vi "Gecko anesthesia specs.vi"(0 "ear folder path":path) -> ()   [LabVIEW 2010]
panel:
  in  "End & don't save":bool
  in  "conc of anesth":string="Concentration of anesthesia delivered (ml/mg): XX"
  in  "tag #":string="Animal number: XX"
  in  "mass":string="Mass (g): XX"
  in  "Length":string="Length (mm): XX"
  in  "method of anesth adminin":string="Method of anesthesia adminisration: XX"
  in  "comments":string="Comments: XX"
  in  "amt of anesth":string="Amount of anesthesia delivered (ml): XX"
  in  "OK; end & save":bool
  in  "anesthetic":string="Anesthetic: XX"
  in  "Sex":string="Sex: XX"
  in  "Animal species":string="Species: XX"
  in  "time of anesth":string="Time of anesthesia administration: XX"
  # "HARD SPECS:"
  # "ANESTHESIA:"
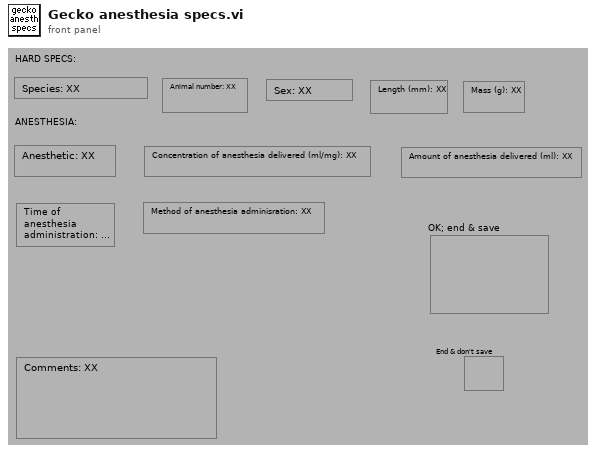
[diagram p1: front panel]
types:
  T1 = cluster{i32, i32, i32, i32, i32, i32, i32, i32, i32}
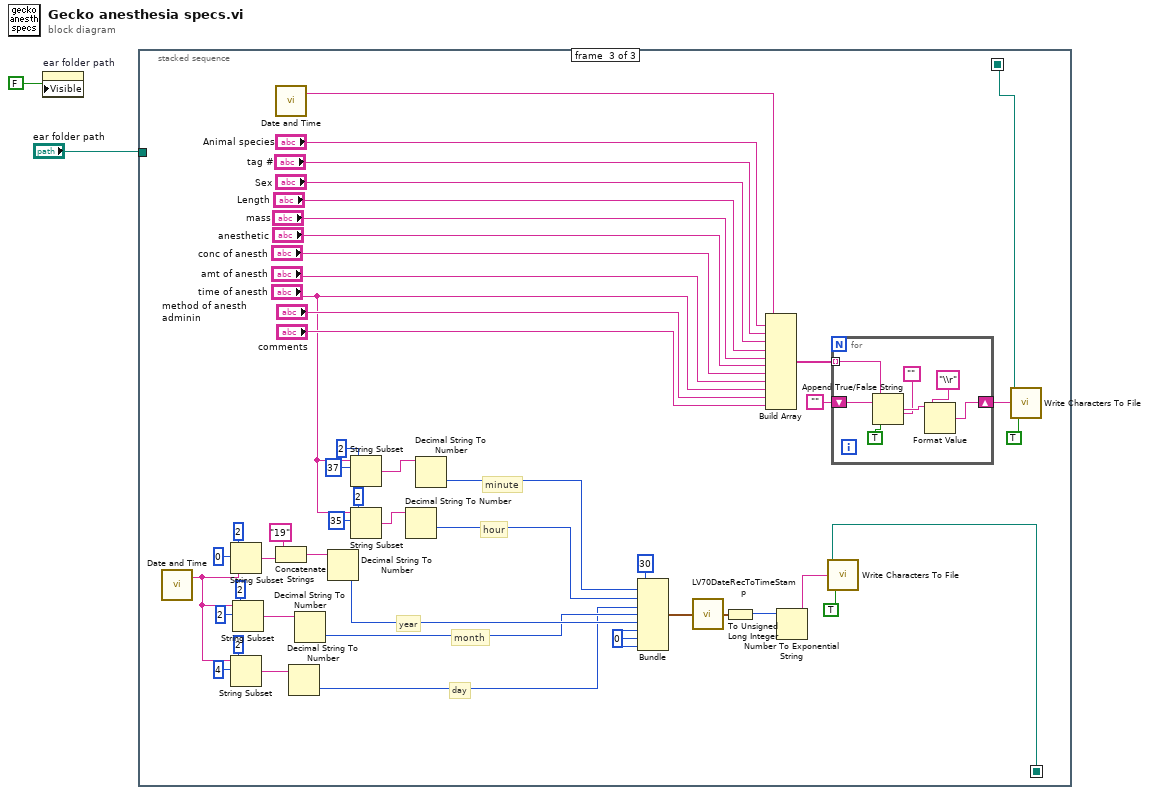
[diagram p0: block diagram]
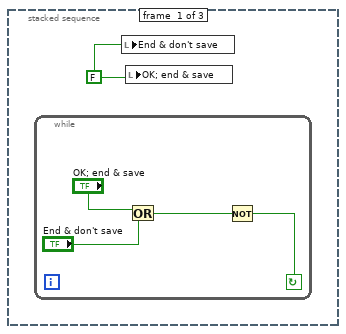
[diagram p2: hidden frame]
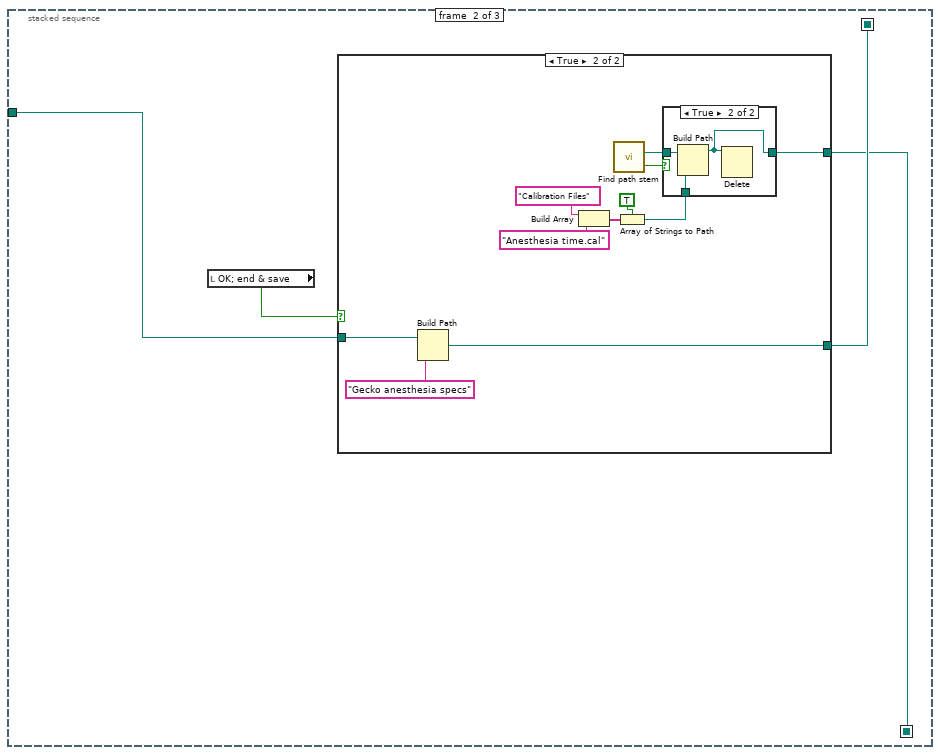
[diagram p3: hidden frame]
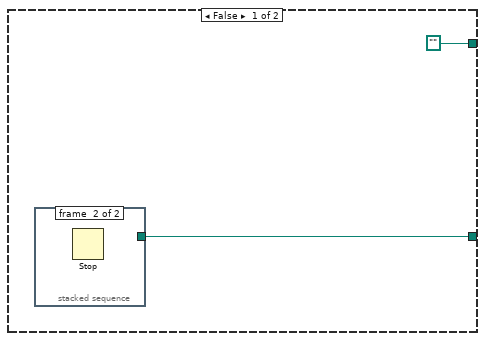
[diagram p4: hidden frame]
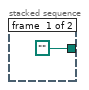
[diagram p5: hidden frame]
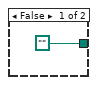
[diagram p6: hidden frame]
diagram:
  n1 = property on="ear folder path" class="Path"("Visible"=FALSE) -> ()  [unwired: 2 in, 2 out]
  n2 = stacked-sequence {
    seq-local: [_ w9 _] -> [_ _ w31]
    seq-local: [_ w8 _] -> [_ _ w34]
    tunnel: "ear folder path" -> [_ w10 _]
    frame #0 {
      w3 = FALSE
      n3 = while {
        stop <- w7 continue-if-true
        n4 = Or(x="OK; end & save", y="End & don't save") -> (x .or. y?=w6:bool)
        n5 = Not(x=w6) -> (.not. x?=w7:bool)
      }
      n6 = local write "End & don't save"(w3) -> ()
      n7 = local write "OK; end & save"(w3) -> ()
    }
    frame #1 {
      n8 = local read "OK; end & save"() -> (w11:bool)
      n9 = case shown="True" w11 {
        tunnel: w10 -> [_ w24]
        tunnel: [w13 w23] -> w9
        tunnel: [path "" w15] -> w8
        frame False {
          n10 = stacked-sequence {
            tunnel: [path "" _] -> w13
            frame #0 {
            }
            frame #1 {
              n11 = Stop() -> ()  [unwired: 1 out]
            }
          }
        }
        frame True {
          n12 = Build Path(base path=w24, name or relative path="Gecko anesthesia specs") -> (appended path=w23:path)
          n13 = Build Array("Calibration Files", "Anesthesia time.cal") -> (w19:string[])
          n14 = call "Find path stem.vi"() -> ("PASS/FAIL"=w17:bool, "Path stem."=w18:path)
          n15 = Array of Strings to Path(0:w19, 1:TRUE) -> (2:w16:path)
          n16 = case shown="True" w17 {
            tunnel: w18 -> [_ w29]
            tunnel: w16 -> [_ w28]
            tunnel: [path "" w27] -> w15
            frame False {
            }
            frame True {
              n17 = Build Path(base path=w29, name or relative path=w28) -> (appended path=w27:path)
              n18 = Delete(path (use dialog)=w27) -> ()  [unwired: 1 in, 6 out]
            }
          }
        }
      }
    }
    frame #2 {
      w55 = 0
      # "day"
      # "month"
      # "year"
      # "hour"
      # "minute"
      n19 = call "Date and Time.vi"() -> ("Date string."=w37:string)  [unwired: 1 out]
      n20 = String Subset(string=w37, offset (0)=0, length (rest)=2) -> (substring=w46:string)
      n21 = String Subset(string=w37, offset (0)=4, length (rest)=2) -> (substring=w36:string)
      n22 = String Subset(string=w37, offset (0)=2, length (rest)=2) -> (substring=w41:string)
      n23 = call "Date and Time.vi"() -> ("Date string."=w75:string)  [unwired: 1 out]
      n24 = Concatenate Strings("19", w46) -> (w45:string)
      n25 = Decimal String To Number(string=w36) -> (number=w35:i32)  [unwired: 3 out]
      n26 = Decimal String To Number(string=w41) -> (number=w40:i32)  [unwired: 3 out]
      n27 = Decimal String To Number(string=w45) -> (number=w44:i32)  [unwired: 3 out]
      n28 = String Subset(string="time of anesth", offset (0)=37, length (rest)=2) -> (substring=w62:string)
      n29 = String Subset(string="time of anesth", offset (0)=35, length (rest)=2) -> (substring=w60:string)
      n30 = Decimal String To Number(string=w60) -> (number=w56:i32)  [unwired: 3 out]
      n31 = Decimal String To Number(string=w62) -> (number=w61:i32)  [unwired: 3 out]
      n32 = Bundle(30, w61, w56, w35, w40, w44, w55, w55, w55) -> (w64:T1)  [unwired: 1 out]
      n33 = call <vilib>:"LV70DateRecToTimeStamp.vi"("date time rec"=w64) -> ("Time Stamp"=w30:timestamp)
      n34 = To Unsigned Long Integer(number=w30) -> (unsigned 32bit integer=w54:u32)
      n35 = Build Array(w75, "Animal species", "tag #", "Sex", "Length", "mass", "anesthetic", "conc of anesth", "amt of anesth", "time of anesth", "method of anesth adminin", "comments") -> (w76:string[])
      n36 = Number To Exponential String(number=w54) -> (E-format string=w65:string)  [unwired: 3 out]
      n37 = call <vilib>:"Write Characters To File.vi"("append to file? (new file:F)"=TRUE, "character string"=w65, "file path (dialog if empty)"=w34) -> ()  [unwired: 3 out]
      n38 = for {
        tunnel: w76 -> [w82] mode=indexing
        shift-right: [w79] -> w32
        shift-left: "" -> [w83]
        n39 = Append True/False String(1:TRUE, 2:"", 3:w82, 4:w83) -> (0:w80:string)
        n40 = Format Value(string ("")=w80, format string="\\r") -> (output string=w79:string)  [unwired: 1 out]
      }
      n41 = call <vilib>:"Write Characters To File.vi"("append to file? (new file:F)"=TRUE, "character string"=w32, "file path (dialog if empty)"=w31) -> ()  [unwired: 3 out]
    }
  }
